vi "Subst Drive.vi"(11 "operation":enum16{"map", "unmap"}(ring)) -> (0 "error out":errorcluster, 2 "standard output":string, 3 "drive":string)   [LabVIEW 2024]
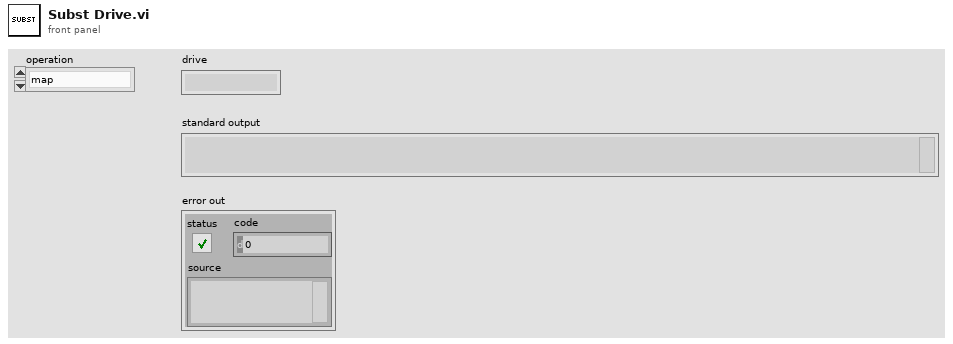
[diagram p1: front panel]
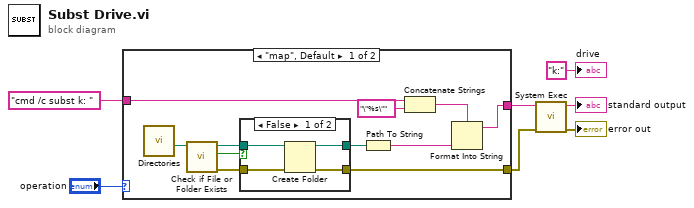
[diagram p0: block diagram]
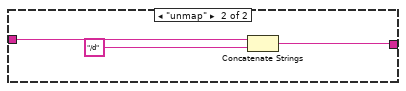
[diagram p3: hidden frame]
diagram:
  n1 = case shown="\"map\", Default" "operation" {
    tunnel: "cmd /c subst k: " -> [w17 w27]
    tunnel: [w14 w25] -> w5
    tunnel: [w8 _] -> w1
    frame "map", Default {
      n2 = call "Directories.vi"() -> ("generated apis"=w13:path)  [unwired: 9 in, 2 out]
      n3 = call <vilib>:"Check if File or Folder Exists.vi"("path"=w13) -> ("error out"=w11:errorcluster, "file or folder exists?"=w12:bool, "dup path"=w10:path)  [unwired: 8 in]
      n4 = case shown="False" w12 {
        tunnel: w11 -> [w22 w23]
        tunnel: w10 -> [w21 w24]
        tunnel: [w20 w24] -> w9
        tunnel: [w19 w23] -> w8
        frame False {
          n5 = Create Folder(path (use dialog)=w21, error in=w22) -> (created path=w20:path, error out=w19:errorcluster)  [unwired: 1 in, 1 out]
        }
        frame True {
        }
      }
      n6 = Path To String(path=w9) -> (string=w18:string)
      n7 = Concatenate Strings(w17, "\"%s\"" ("string")) -> (w15:string)
      n8 = Format Into String(format string=w15, w18) -> (resulting string=w14:string)  [unwired: 2 in, 1 out]
    }
    frame "unmap" {
      n9 = Concatenate Strings(w27, "/d" ("string")) -> (w25:string)
    }
  }
  n10 = call <vilib>:"System Exec.vi"("error in (no error)"=w1, "command line"=w5) -> ("error out"=→"error out":errorcluster, "standard output"=→"standard output":string)  [unwired: 6 in, 2 out]
  "drive" <- "k:" ("drive")
